vi "control_limitLogic.vi"(4 "reinitialize":bool, 6 "limit logic in":bool[](array[boolean]), 7 "dec rate":dbl[](array[numeric]), 8 "diff":dbl, 10 "Previous output":dbl[](array[numeric]), 11 "Desired output":dbl[](array[numeric])) -> (2 "limit logic out":bool[](array[boolean]), 3 "output":dbl[](array[numeric]))   [LabVIEW 2017]
uses:
  <vilib>/addons/control/pid/pid.llb/PID Output Rate Limiter (DBL Array).vi
  <vilib>/addons/control/pid/NI_PID_pid.lvlib
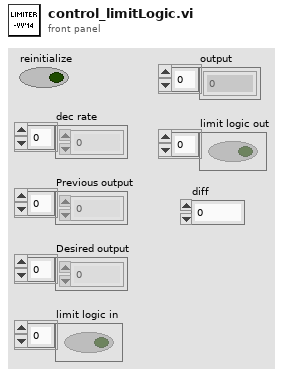
[diagram p1: front panel]
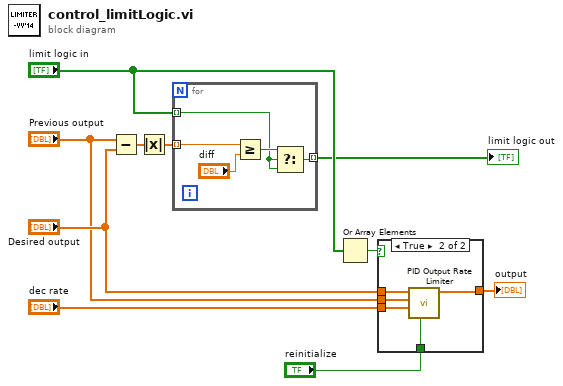
[diagram p0: block diagram]
diagram:
  n1 = Subtract(x="Previous output", y="Desired output") -> (x-y=w3:dbl[])
  n2 = Absolute Value(x=w3) -> (abs(x)=w4:dbl[])
  n3 = for {
    tunnel: w4 -> [w15] mode=indexing
    tunnel: [w14] -> w7 mode=indexing
    tunnel: "limit logic in" -> [w12] mode=indexing
    n4 = Greater Or Equal?(x=w15, y="diff") -> (x >= y?=w13:bool)
    n5 = Select(t=w13, s=w12, f=w12) -> (s? t:f=w14:bool)
  }
  "limit logic out" <- w7
  n6 = Or Array Elements(Boolean array="limit logic in") -> (logical OR=w8:bool)
  n7 = case shown="True" w8 {
    tunnel: "reinitialize" -> [_ w21]
    tunnel: "dec rate" -> [_ w20]
    tunnel: [w16 w19] -> w10
    tunnel: "Previous output" -> [_ w18]
    tunnel: "Desired output" -> [w16 w17]
    frame False {
    }
    frame True {
      n8 = call-poly <vilib>:"PID Output Rate Limiter.vi"("reinitialize? (F)"=w21, "output rate (EGU/min)"=w20, "initial output"=w18, "input (controller output)"=w17) -> ("output"=w19:dbl[])  [unwired: 4 in, 1 out]
    }
  }
  "output" <- w10
